vi "GenerateQueuedCommand.vi"(8 "error in":errorcluster, 11 "T560Channel in":refnum<class "T560Output.lvclass">) -> (0 "error out":errorcluster, 3 "T560Channel out":refnum<class "T560Output.lvclass">)   [LabVIEW 2020, in "T560Output.lvclass"]
uses:
  T560Output.lvclass
  C:/GEECS/Developers Version/source/Device Drivers/Highland T564 DDG/SupportLibraries/DeviceSpecific/HighlandT560Lib/T560ChannelClass/T560Channel.lvclass
  T560Output.lvclass/T560Output.ctl
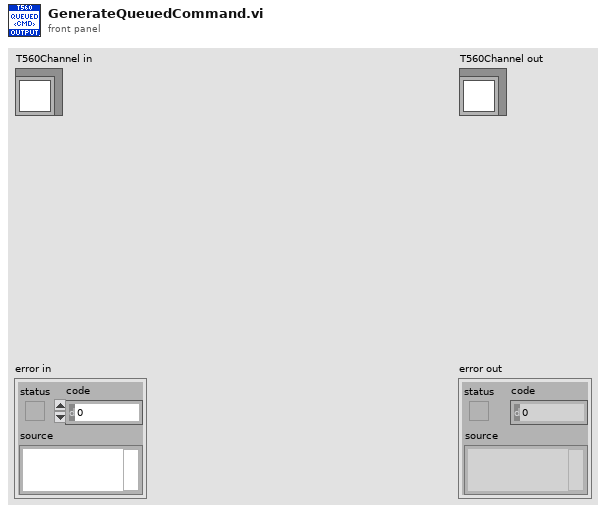
[diagram p1: front panel]
types:
  T1 = typedef "Highlandt564.lvlib/T560Channel.lvclass/ChannelName.ctl" = enum16{"Null", "A", "B", "C", "D", "Trigger"}
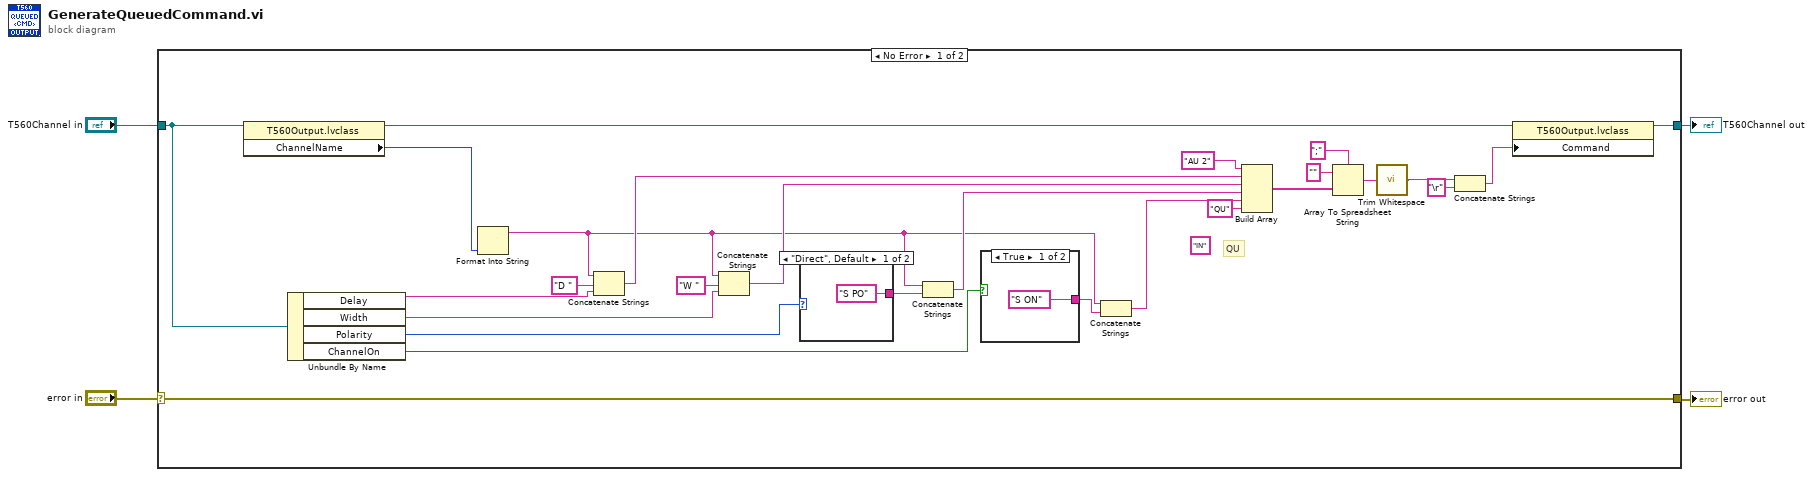
[diagram p0: block diagram]
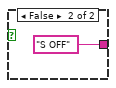
[diagram p2: hidden frame]
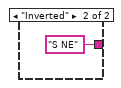
[diagram p3: hidden frame]
diagram:
  n1 = case shown="No Error" "error in" {
    selector: "error in" -> [w6 w37]
    tunnel: "T560Channel in" -> [w8 w36]
    tunnel: [w6 w37] -> w4
    tunnel: [w10 w36] -> w3
    frame No Error {
      (unwired) "IN" ("element")
      # "QU"
      n2 = property class="T560Output.lvclass"(reference=w8) -> (reference out=w7:refnum<class "T560Output.lvclass">, "ChannelName"=w9:T1)  [unwired: 1 in, 1 out]
      n3 = Unbundle By Name(w8) -> ("Delay"=w18:string, "Width"=w31:string, "Polarity"=w20:enum16{"Direct", "Inverted"}, "ChannelOn"=w22:bool)
      n4 = Format Into String(w9) -> (resulting string=w15:string)  [unwired: 3 in, 1 out]
      n5 = Concatenate Strings(w15, "D ", w18) -> (w26:string)
      n6 = Concatenate Strings(w15, "W ", w31) -> (w27:string)
      n7 = case shown="\"Direct\", Default" w20 {
        tunnel: ["S PO" "S NE"] -> w19
        frame "Direct", Default {
        }
        frame "Inverted" {
        }
      }
      n8 = Concatenate Strings(w15, w19) -> (w21:string)
      n9 = case shown="True" w22 {
        tunnel: ["S ON" "S OFF"] -> w23
        frame True {
        }
        frame False {
        }
      }
      n10 = Concatenate Strings(w15, w23) -> (w24:string)
      n11 = Build Array("AU 2" ("element"), w26, w27, w21, w24, "QU" ("element")) -> (w28:string[])
      n12 = Array To Spreadsheet String(delimiter (Tab)=";", array=w28, 3:"" ("format string")) -> (spreadsheet string=w13:string)
      n13 = call "Trim Whitespace.vi"("string"=w13) -> ("trimmed string"=w12:string)  [unwired: 1 in]
      n14 = Concatenate Strings(w12, "\r" ("string")) -> (w11:string)
      n15 = property class="T560Output.lvclass"(reference=w7, "Command"=w11) -> (reference out=w10:refnum<class "T560Output.lvclass">)  [unwired: 1 in, 1 out]
    }
    frame Error {
    }
  }
  "error out" <- w4
  "T560Channel out" <- w3
